vi "Write to DB.vi"(8 "error in (no error)":errorcluster, 11 "Database Entry in":refnum<class "Database Entry.lvclass">) -> (0 "error out":errorcluster, 2 "Stack names":string[](array[string]), 3 "Database Entry out":refnum<class "Database Entry.lvclass">)   [LabVIEW 2021, in "Database Entry.lvclass"]
uses:
  Database Entry.lvclass
  Database Entry.lvclass/Database Entry.ctl
  <vilib>/Utility/file.llb/Read Delimited Spreadsheet (string).vi
  <vilib>/Utility/file.llb/Write Delimited Spreadsheet (string).vi
  Components/Stack/Stack.lvclass
panel:
  out "Final name":string
  out "Data cluster":T1={"module or proto"="proto", " geometry"="full", "resolution"="LD", "baselayer"="BA_123", "toplayer"="SI_789", "bl_pos"="1", "tl_pos"="1", "put_pos"="1", "region"="1", "asstray"="1", "comptray"="1", "put"="1", "date"="2024-04-02", "timestart"="1:12:12.442", "timeend"="1:23:45.244", "operator"="cmuperson", "tape"="some", "glue"="some", "stack name"="some", "Adhesive type"="", "Comments"="", "Temperature"="", "Relative Humidity"="", "Sensor grade"="", "ROC version"="", "Baseplate material"=""}
  out "error out py":errorcluster
  out "String Out":string="Upload Success"
  in  "error in (no error) py":errorcluster
  # "Debug instructions\n#### The order of values in db_data_cols must match the order of values in Data cluster in Stack.lvclass: Get stack data.vi \n#### The variable names below correspond to postgres col name. LV does not neet to match the col numes but just the values. \n#### Right-click on the Data cluster on the front panel and click on 'reorder controls' to verify the order is correct in the code. \n#### The physical position of the fields is different from the actual position.\n\nIn Main VIs/python_db/postgres_tools.py, see functions 'assembly_data' and 'assembly_data_as_list'."
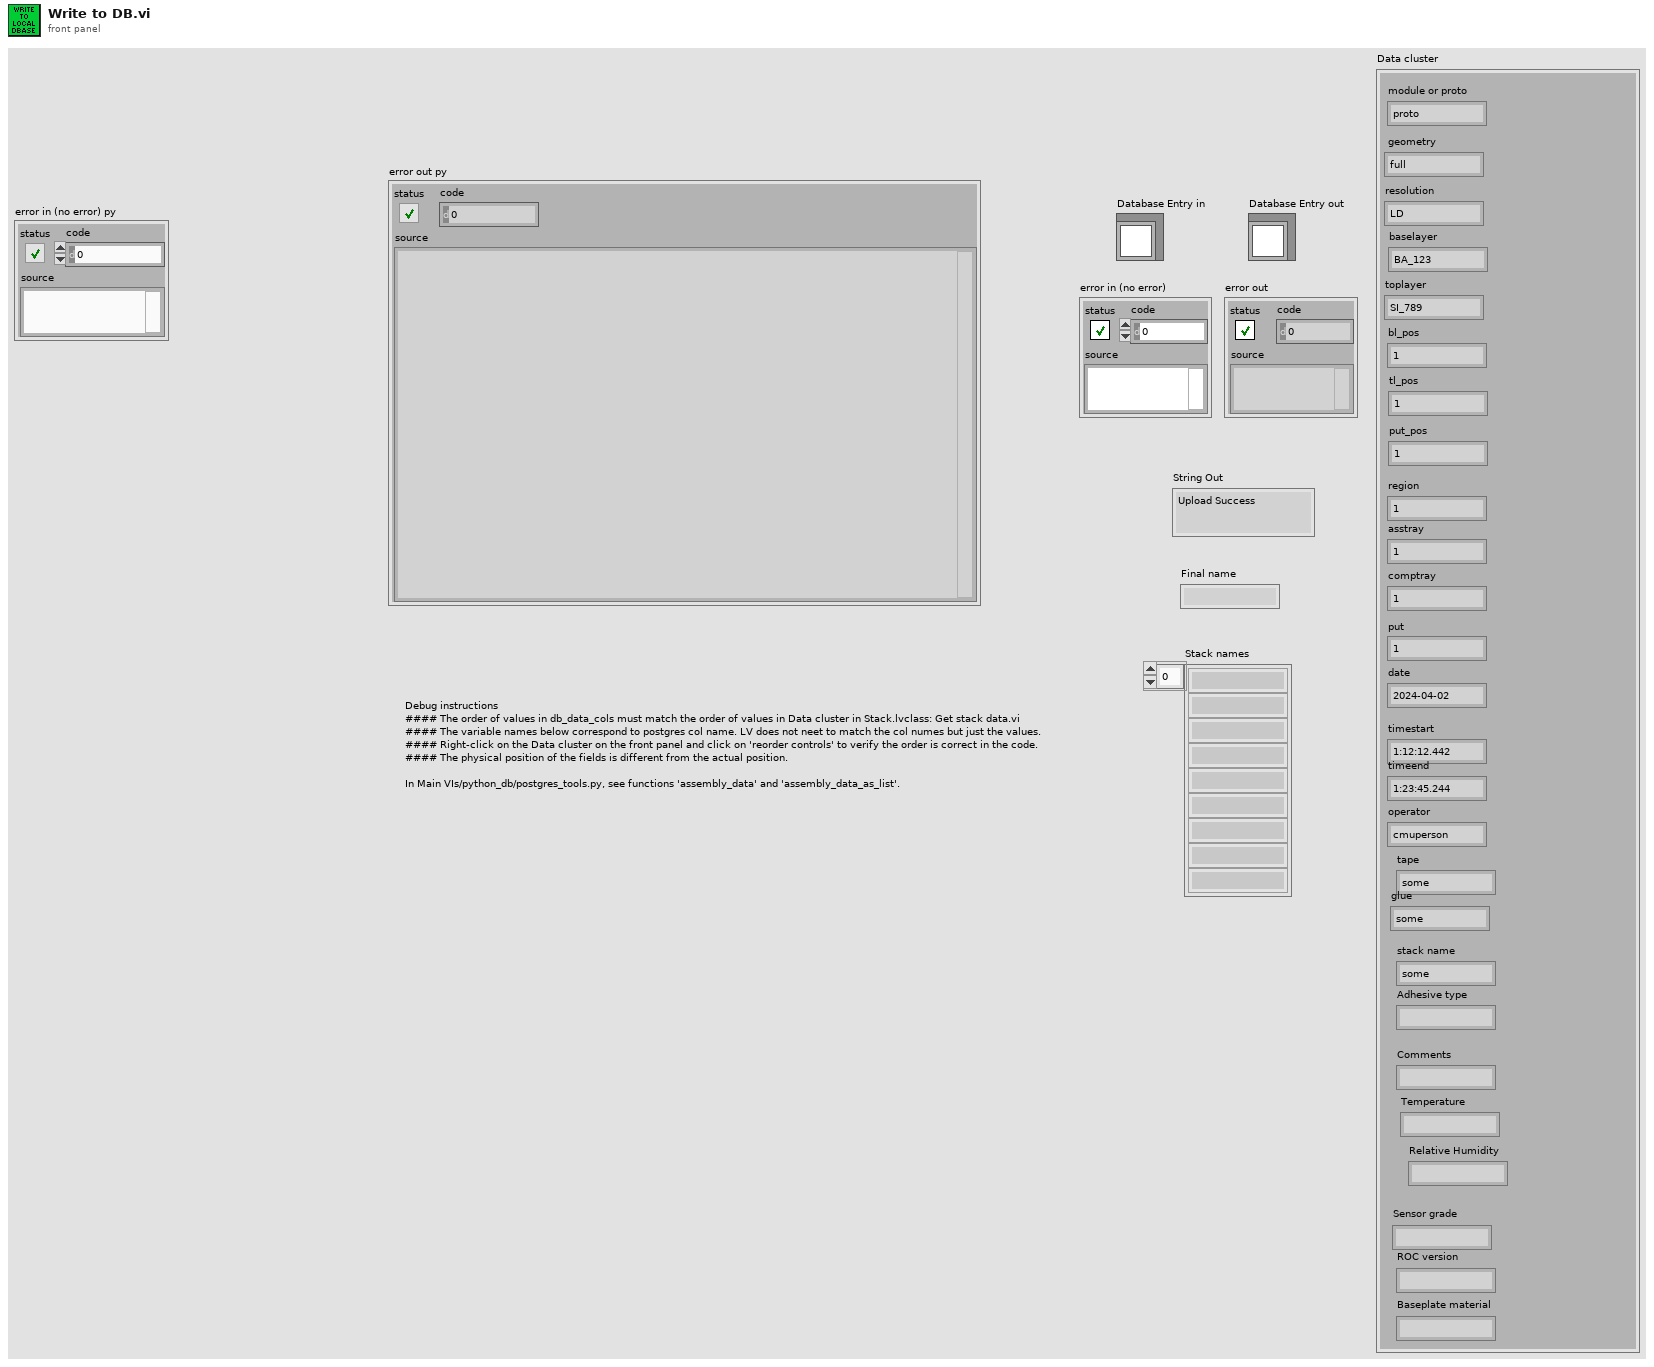
[diagram p1: front panel]
types:
  T1 = cluster{"module or proto":string, " geometry":string, "resolution":string, "baselayer":string, "toplayer":string, "bl_pos":string, "tl_pos":string, "put_pos":string, "region":string, "asstray":string, "comptray":string, "put":string, "date":string, "timestart":string, "timeend":string, "operator":string, "tape":string, "glue":string, "stack name":string, "Adhesive type":string, "Comments":string, "Temperature":string, "Relative Humidity":string, "Sensor grade":string, "ROC version":string, "Baseplate material":string}
  T2 = typedef "File Paths.ctl" = cluster{"Glue Pattern Folder":path, "Carrier Tray Folder":path, "Pick Up Tool Fixture Folder":path, "Components Folder":path, "Bellows Tool Offset.txt":path, "Pick Up Tool Offset.txt":path, "Dispense Tip Offset.txt":path, "Log Files":path, "Gantry Assembly Map.txt":path, "Syringe and offset map.txt":path, "Controllers Folder":path, "Local dbase config":path}
  T3 = cluster{"type (proto/module)":string, " geometry":string, "resolution":string, "baselayer":string, "toplayer":string, "bl_pos":string, "tl_pos":string, "put_pos":string, "region":string, "asstray":string, "comptray":string, "put":string, "date":string, "timestart":string, "timeend":string, "operator":string, "tape":string, "glue":string, "stack name":string, "Adhesive type":string, "Comments":string, "Temperature":string, "Relative Humidity":string, "Sensor grade":string, "ROC version":string, "Baseplate material":string}
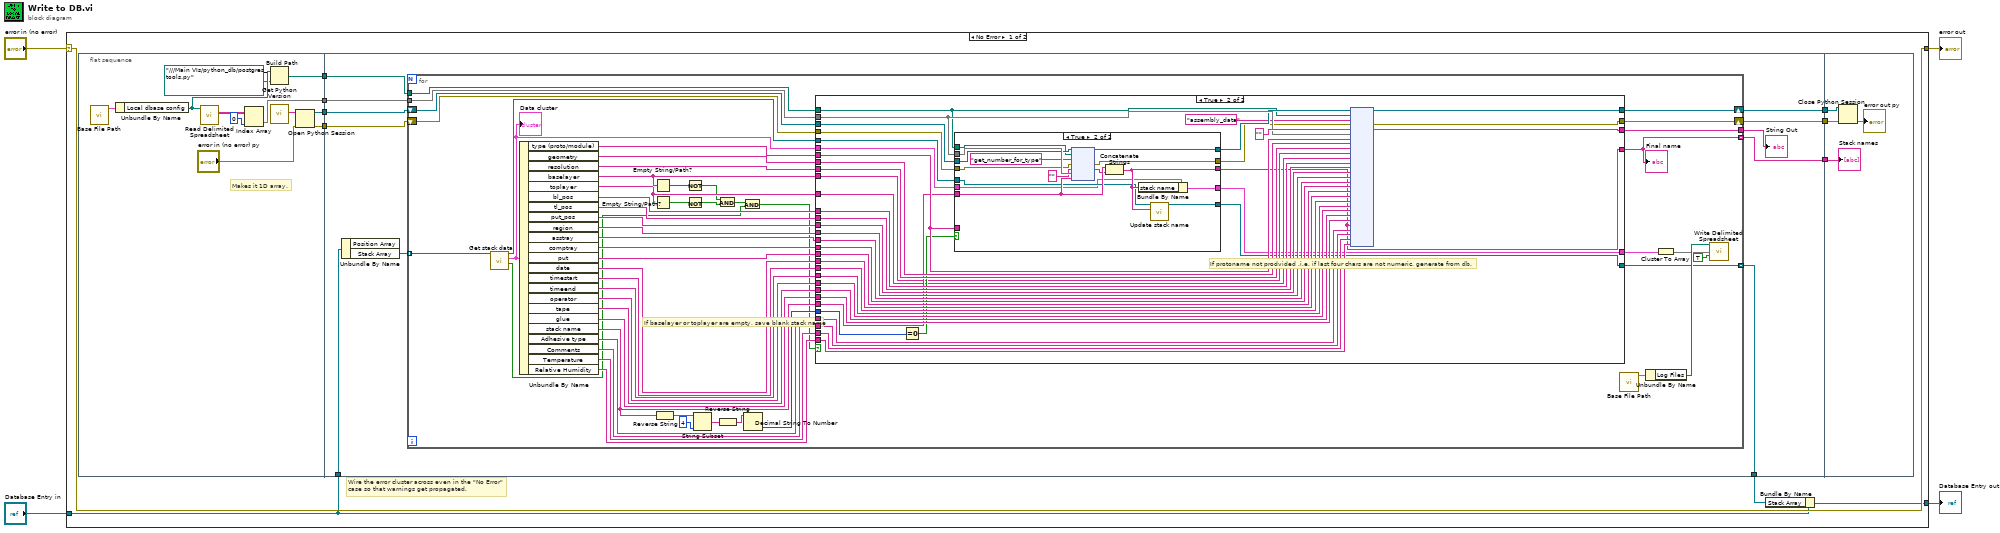
[diagram p0: block diagram]
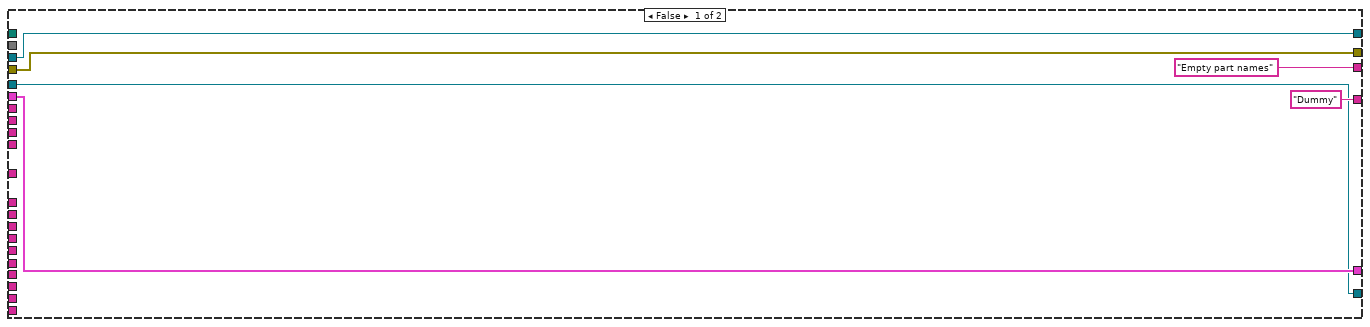
[diagram p2: hidden frame]
diagram:
  n1 = case shown="No Error" "error in (no error)" {
    selector: "error in (no error)" -> [w15 w162]
    tunnel: [w15 w162] -> w3
    tunnel: [w7 w161] -> w1
    tunnel: "Database Entry in" -> [w6 w161]
    frame No Error {
      # "Wire the error cluster across even in the \"No Error\"\ncase so that warnings get propagated."
      n2 = flat-sequence {
        tunnel: [w25] -> w14
        tunnel: [w26] -> w13
        tunnel: [w22] -> w12
        tunnel: [w18] -> w11
        tunnel: [w36] -> w10
        tunnel: [w35] -> w9
        tunnel: w14 -> [w37]
        tunnel: w13 -> [w34]
        tunnel: w12 -> [w33]
        tunnel: w11 -> [w32]
        tunnel: w6 -> [w31]
        tunnel: [w28] -> w8
        tunnel: [w27] -> w5
        tunnel: w10 -> [w159]
        tunnel: w9 -> [w160]
        tunnel: w8 -> [w157]
        frame #0 {
          # "Makes it 1D array."
          n3 = call "Base File Path.vi"() -> ("Paths Out"=w23:T2)  [unwired: 11 in]
          n4 = Unbundle By Name(w23) -> ("Local dbase config"=w21:path)
          n5 = call-poly <vilib>:"Read Delimited Spreadsheet.vi"("file path (dialog if empty)"=w21) -> ("all rows"=w20:string[][])  [unwired: 9 in, 5 out]
          n6 = Index Array(array=w20, index (col)=0 ("disabled index (col)")) -> (element=w18:string[])  [unwired: 1 in]
          n7 = Build Path(base path=w21, name or relative path=path "../../../Main VIs/python_db/postgres_tools.py" ("module path")) -> (appended path=w22:path)
          n8 = call "Get Python Version.vi"() -> ("Python Version"=w16:string)  [unwired: 10 in, 1 out]
          n9 = Open Python Session(python version=w16, 3:"error in (no error) py") -> (session out=w26:refnum<k35>, error out=w25:errorcluster)  [unwired: 1 in]
        }
        frame #1 {
          n10 = Unbundle By Name(w31) -> ("Stack Array"=w29:refnum<class "Stack.lvclass">[])  [unwired: 1 out]
          n11 = for {
            tunnel: w33 -> [w66]
            shift-right: [w89] -> w36
            shift-left: w37 -> [w65]
            shift-right: [w88] -> w35
            shift-left: w34 -> [w67]
            tunnel: [w87] -> w30
            tunnel: w29 -> [w86] mode=indexing
            tunnel: w32 -> [w68]
            tunnel: [w53] -> w28 mode=indexing
            tunnel: [w45] -> w27 mode=indexing
            # "If baselayer or toplayer are empty, save blank stack name"
            n12 = call "Get stack data.vi"("Stack in"=w86) -> ("Is real run"=w38:bool, "Data cluster"=w48:T3, "Stack out"=w46:refnum<class "Stack.lvclass">)  [unwired: 7 in, 1 out]
            "Data cluster" <- w48
            n13 = Unbundle By Name(w48) -> ("type (proto/module)"=w69:string, "geometry"=w85:string, "resolution"=w84:string, "baselayer"=w55:string, "toplayer"=w54:string, "bl_pos"=w83:string, "tl_pos"=w82:string, "put_pos"=w81:string, "region"=w64:string, "asstray"=w80:string, "comptray"=w79:string, "put"=w78:string, "date"=w77:string, "timestart"=w76:string, "timeend"=w75:string, "operator"=w74:string, "tape"=w73:string, "glue"=w72:string, "stack name"=w56:string, "Adhesive type"=w63:string, "Comments"=w62:string, "Temperature"=w52:string, "Relative Humidity"=w51:string)
            n14 = Empty String/Path?(string/path=w55) -> (empty?=w44:bool)
            n15 = Empty String/Path?(string/path=w54) -> (empty?=w43:bool)
            n16 = Reverse String(1:w56) -> (0:w61:string)
            n17 = Not(x=w44) -> (.not. x?=w42:bool)
            n18 = Not(x=w43) -> (.not. x?=w41:bool)
            n19 = String Subset(string=w61, length (rest)=4 ("length (rest)")) -> (substring=w59:string)  [unwired: 1 in]
            n20 = And(x=w42, y=w41) -> (x .and. y?=w40:bool)
            n21 = Reverse String(1:w59) -> (0:w58:string)
            n22 = And(x=w40, y=w38) -> (x .and. y?=w39:bool)
            n23 = Decimal String To Number(string=w58) -> (number=w57:i32)  [unwired: 2 in, 1 out]
            n24 = case shown="True" w39 {
              tunnel: [w94 w136] -> w89
              tunnel: [w95 w135] -> w88
              tunnel: ["Empty part names" w134] -> w87
              tunnel: w85 -> [_ w132]
              tunnel: w84 -> [_ w131]
              tunnel: w83 -> [_ w130]
              tunnel: w82 -> [_ w129]
              tunnel: w81 -> [_ w128]
              tunnel: w80 -> [_ w127]
              tunnel: w79 -> [_ w126]
              tunnel: w78 -> [_ w125]
              tunnel: w77 -> [_ w124]
              tunnel: w76 -> [_ w123]
              tunnel: w75 -> [_ w122]
              tunnel: w74 -> [_ w121]
              tunnel: w73 -> [_ w120]
              tunnel: w72 -> [_ w119]
              tunnel: w69 -> [_ w118]
              tunnel: w68 -> [_ w117]
              tunnel: w67 -> [w95 w116]
              tunnel: w66 -> [_ w114]
              tunnel: w65 -> [w94 w113]
              tunnel: w64 -> [_ w110]
              tunnel: w63 -> [_ w109]
              tunnel: w62 -> [_ w108]
              tunnel: w57 -> [_ w107]
              tunnel: w56 -> [_ w106]
              tunnel: w55 -> [_ w104]
              tunnel: w54 -> [_ w103]
              tunnel: ["Dummy" ("stack name") w100] -> w53
              tunnel: w52 -> [_ w102]
              tunnel: w51 -> [_ w101]
              tunnel: w48 -> [w91 w97]
              tunnel: [w91 w96] -> w47
              tunnel: w46 -> [w90 w98]
              tunnel: [w90 w99] -> w45
              frame False {
              }
              frame True {
                # "If protoname not prodvided ,i.e. if last four chars are not numeric, generate from db."
                n25 = Equal To 0?(x=w107) -> (x = 0?=w105:bool)
                n26 = case shown="True" w105 {
                  tunnel: w118 -> [_ _]
                  tunnel: w106 -> [w139 w156]
                  tunnel: w117 -> [_ w155]
                  tunnel: w116 -> [w141 w154]
                  tunnel: [w141 w153] -> w115
                  tunnel: w114 -> [_ w152]
                  tunnel: w113 -> [w140 w151]
                  tunnel: [w140 w150] -> w112
                  tunnel: [w139 w149] -> w100
                  tunnel: [w138 w145] -> w99
                  tunnel: w98 -> [w138 w144]
                  tunnel: w97 -> [w137 w143]
                  tunnel: [w137 w142] -> w96
                  frame False {
                  }
                  frame True {
                    n27 = node(w154, w152, "get_number_for_type" ("function name"), w151, "" ("function name"), w155, w156) -> (w153:refnum<k35>, w150:errorcluster, w146:string)  [unwired: 2 in, 2 out]
                    n28 = Concatenate Strings(w156, w146) -> (w149:string)
                    n29 = Bundle By Name(cluster=w143, "stack name"=w149) -> (w142:T3)
                    n30 = call "Update stack name.vi"("Stack ID updated"=w149, "Stack in"=w144) -> ("Stack out"=w145:refnum<class "Stack.lvclass">)  [unwired: 8 in, 1 out]
                  }
                }
                n31 = node(w115, w114, "assembly_data" ("function name"), w112, "", w117, w118, w132, w131, w104, w103, w130, w129, w128, w110, w127, w126, w125, w124, w123, w122, w121, w120, w119, w100, w109, w108, w102, w101) -> (w135:refnum<k35>, w136:errorcluster, w134:string)  [unwired: 24 in, 2 out]
              }
            }
            "Final name" <- w53
            n32 = call "Base File Path.vi"() -> ("Paths Out"=w71:T2)  [unwired: 11 in]
            n33 = Unbundle By Name(w71) -> ("Log Files"=w70:path)
            n34 = Cluster To Array(cluster=w47) -> (array=w49:string[])
            n35 = call-poly <vilib>:"Write Delimited Spreadsheet.vi"("file path (dialog if empty)"=w70, "1D data"=w49, "append to file? (new file:F)"=TRUE) -> ()  [unwired: 11 in, 2 out]
          }
          "String Out" <- w30
        }
        frame #2 {
          n36 = Close Python Session(session in=w160, error in=w159) -> (11:→"error out py":errorcluster)
          "Stack names" <- w157
        }
      }
      n37 = Bundle By Name(cluster=w6, "Stack Array"=w5) -> (w7:refnum<class "Database Entry.lvclass">)
    }
    frame Error {
    }
  }
  "error out" <- w3
  "Database Entry out" <- w1
